vi "NEW_Surge IFSM.vi"() -> ()   [LabVIEW 2019]
uses:
  <vilib>/Utility/NIReport.llb/Report Type.ctl
  <vilib>/Utility/NIReport.llb/NI_report.lvclass
  <vilib>/Utility/NIReport.llb/NI_ReportGenerationCore.lvlib
  <vilib>/Utility/NIReport.llb/Excel/NI_Excel.lvclass
panel:
  in  "REQUEST NUMBER":i32
  out "STEP 8":bool
  out "STEP 7":bool
  out "STEP 6":bool
  out "STEP 5":bool
  in  "START Button":bool
  out "STEP 4":bool
  out "STEP 3":bool
  out "STEP 2":bool
  out "STEP 1":bool
  in  "FILE PATH":path
  # "DATA SUMMARY FOR SURGE IFSM"
  # "OPEN EXCEL FILE"
  # "RUN MACRO INTO EXCEL FILE"
  # "Create New Sheet named (Request Number_Surge_IFSM)"
  # "Create Table named (\"Last  Good Pass\")"
  # "Create New Sheet and Table named (\"Summary Table\")"
  # "Move All Tabs into a new Excel Workbook"
  # "SAVE EXCEL FILE"
  # "FINISH"
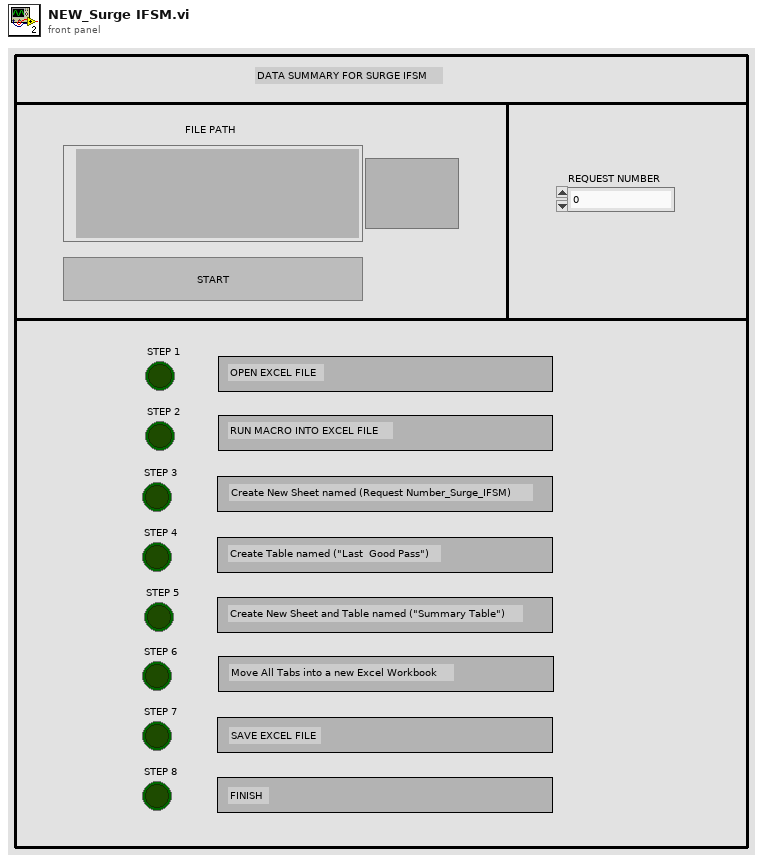
[diagram p1: front panel]
types:
  T1 = enum16{"maximized", "minimized", "normal", "no change"}
  T2 = typedef "NI_ReportGenerationCore.lvlib/Report Type.ctl" = enum16{"HTML", "Word", "Excel"}
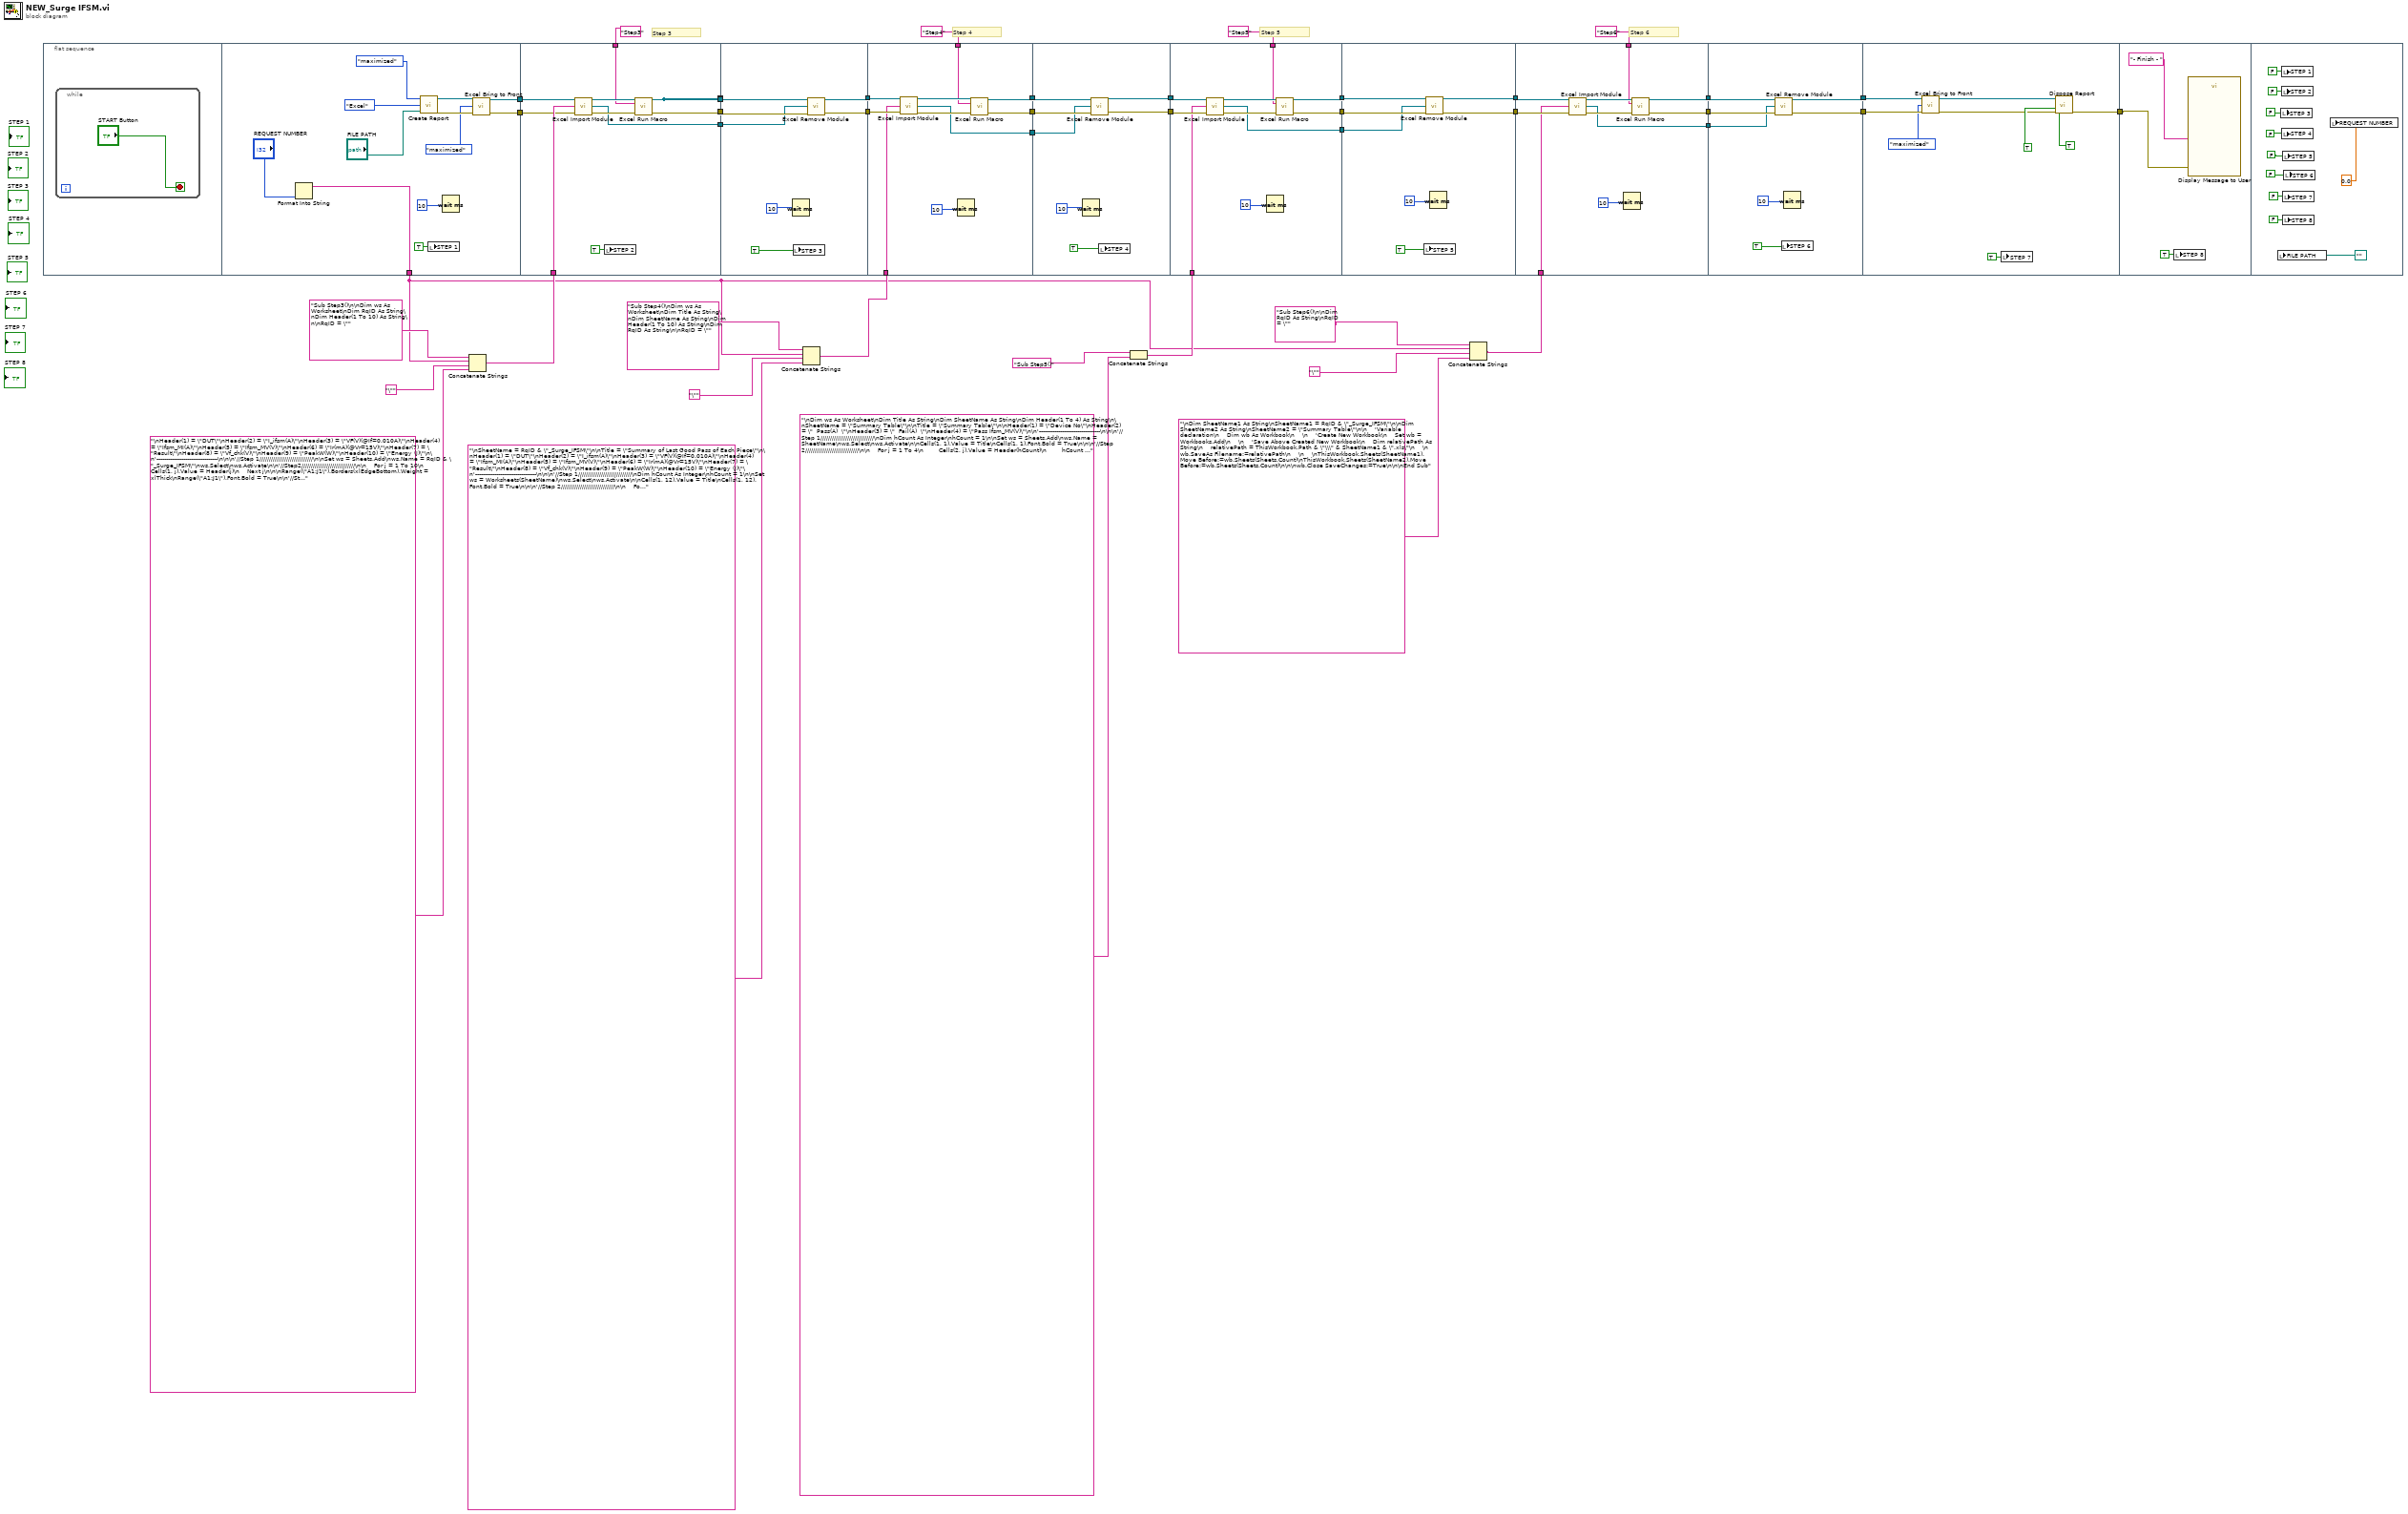
[diagram p0: block diagram]
diagram:
  # "Step 3"
  # "Step 6"
  # "Step 5"
  # "Step 4"
  n1 = flat-sequence {
    tunnel: [w50] -> w38
    tunnel: [w49] -> w37
    tunnel: [w46] -> w1
    tunnel: [w65] -> w43
    tunnel: [w63] -> w42
    tunnel: "Step3" ("macro name") -> [w64]
    tunnel: [w63] -> w40
    tunnel: [w62] -> w39
    tunnel: w20 -> [w60]
    tunnel: w38 -> [w59]
    tunnel: w37 -> [w58]
    tunnel: w43 -> [w73]
    tunnel: [w71] -> w36
    tunnel: w42 -> [_]
    tunnel: [w72] -> w35
    tunnel: w40 -> [w74]
    tunnel: w39 -> [w70]
    tunnel: w36 -> [w81]
    tunnel: [w79] -> w34
    tunnel: w35 -> [w84]
    tunnel: [w82] -> w33
    tunnel: "Step4" ("macro name") -> [w78]
    tunnel: [w77] -> w21
    tunnel: w3 -> [w76]
    tunnel: w34 -> [w90]
    tunnel: w33 -> [w87]
    tunnel: [w89] -> w23
    tunnel: [w88] -> w22
    tunnel: w21 -> [w86]
    tunnel: [w96] -> w32
    tunnel: [w99] -> w31
    tunnel: w23 -> [w98]
    tunnel: w22 -> [w101]
    tunnel: "Step5" ("macro name") -> [w95]
    tunnel: [w94] -> w18
    tunnel: w17 -> [w93]
    tunnel: w32 -> [w107]
    tunnel: [w106] -> w28
    tunnel: w31 -> [w104]
    tunnel: [w105] -> w26
    tunnel: w18 -> [w103]
    tunnel: w28 -> [w118]
    tunnel: [w116] -> w27
    tunnel: w26 -> [w115]
    tunnel: [w113] -> w25
    tunnel: "Step6" ("macro name") -> [w112]
    tunnel: [w111] -> w15
    tunnel: w14 -> [w110]
    tunnel: w27 -> [w124]
    tunnel: [w123] -> w30
    tunnel: w25 -> [w122]
    tunnel: [w121] -> w29
    tunnel: w15 -> [w120]
    tunnel: w30 -> [w129]
    tunnel: w29 -> [w130]
    tunnel: [w133] -> w44
    tunnel: w44 -> [w135]
    frame #0 {
      n2 = while {
        stop <- "START Button" stop-if-true
      }
    }
    frame #1 {
      n3 = Format Into String("REQUEST NUMBER") -> (resulting string=w46:string)  [unwired: 3 in, 1 out]
      n4 = call <vilib>:"Create Report.vi"("window state (normal)"=T1."maximized", "report type"=Report_Type."Excel", "template (empty)"="FILE PATH") -> ("report out"=w53:refnum<class "NI_report.lvclass">, "error out"=w54:errorcluster)  [unwired: 11 in]
      n5 = local write "STEP 1"(TRUE ("STEP 1")) -> ()
      n6 = Wait (ms)(milliseconds to wait=u32 10 ("millisecond timer value")) -> ()  [unwired: 1 out]
      n7 = call <vilib>:"Excel Bring to Front.vi"("report in"=w53, "window state (maximized)"=enum16{"maximized", "minimized", "normal"}."maximized", "error in (no error)"=w54) -> ("report out"=w50:refnum<class "NI_report.lvclass">, "error out"=w49:errorcluster)  [unwired: 11 in]
    }
    frame #2 {
      n8 = call <vilib>:"Excel Import Module.vi"("report in"=w59, "module code (\"\")"=w60, "error in (no error)"=w58) -> ("report out"=w67:refnum<class "NI_report.lvclass">, "module reference"=w62:refnum<k7>, "error out"=w66:errorcluster)  [unwired: 10 in]
      n9 = local write "STEP 2"(TRUE ("STEP 2")) -> ()
      n10 = call <vilib>:"Excel Run Macro.vi"("report in"=w67, "macro name"=w64, "error in (no error)"=w66) -> ("report out"=w63:refnum<class "NI_report.lvclass">, "error out"=w65:errorcluster)  [unwired: 10 in, 1 out]
    }
    frame #3 {
      n11 = Wait (ms)(milliseconds to wait=u32 10 ("millisecond timer value")) -> ()  [unwired: 1 out]
      n12 = local write "STEP 3"(TRUE) -> ()
      n13 = call <vilib>:"Excel Remove Module.vi"("report in"=w74, "module reference"=w70, "error in (no error)"=w73) -> ("report out"=w72:refnum<class "NI_report.lvclass">, "error out"=w71:errorcluster)  [unwired: 11 in]
    }
    frame #4 {
      n14 = call <vilib>:"Excel Import Module.vi"("report in"=w84, "module code (\"\")"=w76, "error in (no error)"=w81) -> ("report out"=w83:refnum<class "NI_report.lvclass">, "module reference"=w77:refnum<k7>, "error out"=w80:errorcluster)  [unwired: 10 in]
      n15 = Wait (ms)(milliseconds to wait=u32 10 ("millisecond timer value")) -> ()  [unwired: 1 out]
      n16 = call <vilib>:"Excel Run Macro.vi"("report in"=w83, "macro name"=w78, "error in (no error)"=w80) -> ("report out"=w82:refnum<class "NI_report.lvclass">, "error out"=w79:errorcluster)  [unwired: 10 in, 1 out]
    }
    frame #5 {
      n17 = Wait (ms)(milliseconds to wait=u32 10 ("millisecond timer value")) -> ()  [unwired: 1 out]
      n18 = call <vilib>:"Excel Remove Module.vi"("report in"=w87, "module reference"=w86, "error in (no error)"=w90) -> ("report out"=w88:refnum<class "NI_report.lvclass">, "error out"=w89:errorcluster)  [unwired: 11 in]
      n19 = local write "STEP 4"(TRUE) -> ()
    }
    frame #6 {
      n20 = call <vilib>:"Excel Import Module.vi"("report in"=w101, "module code (\"\")"=w93, "error in (no error)"=w98) -> ("report out"=w100:refnum<class "NI_report.lvclass">, "module reference"=w94:refnum<k7>, "error out"=w97:errorcluster)  [unwired: 10 in]
      n21 = Wait (ms)(milliseconds to wait=u32 10 ("millisecond timer value")) -> ()  [unwired: 1 out]
      n22 = call <vilib>:"Excel Run Macro.vi"("report in"=w100, "macro name"=w95, "error in (no error)"=w97) -> ("report out"=w99:refnum<class "NI_report.lvclass">, "error out"=w96:errorcluster)  [unwired: 10 in, 1 out]
    }
    frame #7 {
      n23 = local write "STEP 5"(TRUE) -> ()
      n24 = call <vilib>:"Excel Remove Module.vi"("report in"=w104, "module reference"=w103, "error in (no error)"=w107) -> ("report out"=w105:refnum<class "NI_report.lvclass">, "error out"=w106:errorcluster)  [unwired: 11 in]
      n25 = Wait (ms)(milliseconds to wait=u32 10 ("millisecond timer value")) -> ()  [unwired: 1 out]
    }
    frame #8 {
      n26 = call <vilib>:"Excel Import Module.vi"("report in"=w115, "module code (\"\")"=w110, "error in (no error)"=w118) -> ("report out"=w114:refnum<class "NI_report.lvclass">, "module reference"=w111:refnum<k7>, "error out"=w117:errorcluster)  [unwired: 10 in]
      n27 = Wait (ms)(milliseconds to wait=u32 10 ("millisecond timer value")) -> ()  [unwired: 1 out]
      n28 = call <vilib>:"Excel Run Macro.vi"("report in"=w114, "macro name"=w112, "error in (no error)"=w117) -> ("report out"=w113:refnum<class "NI_report.lvclass">, "error out"=w116:errorcluster)  [unwired: 10 in, 1 out]
    }
    frame #9 {
      n29 = call <vilib>:"Excel Remove Module.vi"("report in"=w122, "module reference"=w120, "error in (no error)"=w124) -> ("report out"=w121:refnum<class "NI_report.lvclass">, "error out"=w123:errorcluster)  [unwired: 11 in]
      n30 = local write "STEP 6"(TRUE) -> ()
      n31 = Wait (ms)(milliseconds to wait=u32 10 ("millisecond timer value")) -> ()  [unwired: 1 out]
    }
    frame #10 {
      n32 = call <vilib>:"Excel Bring to Front.vi"("report in"=w130, "window state (maximized)"=enum16{"maximized", "minimized", "normal"}."maximized", "error in (no error)"=w129) -> ("report out"=w127:refnum<class "NI_report.lvclass">, "error out"=w126:errorcluster)  [unwired: 11 in]
      n33 = local write "STEP 7"(TRUE ("STEP 3")) -> ()
      n34 = call-dynamic "Dispose Report.vi"("report in"=w127, "save changes? (F)"=TRUE, "error in (no error)"=w126, "close report? (T)"=TRUE) -> ("error out"=w133:errorcluster)  [unwired: 11 in]
    }
    frame #11 {
      n35 = local write "STEP 8"(TRUE ("STEP 4")) -> ()
      n36 = call "Display Message to User"("error in (no error)"=w135, "Message"="- Finish - ") -> ()  [unwired: 8 in, 2 out]
    }
    frame #12 {
      n37 = local write "FILE PATH"(path "" ("FILE PATH")) -> ()
      n38 = local write "STEP 3"(FALSE) -> ()
      n39 = local write "STEP 1"(FALSE ("STEP 1")) -> ()
      n40 = local write "STEP 2"(FALSE ("STEP 2")) -> ()
      n41 = local write "STEP 4"(FALSE) -> ()
      n42 = local write "STEP 5"(FALSE) -> ()
      n43 = local write "STEP 7"(FALSE ("STEP 3")) -> ()
      n44 = local write "STEP 8"(FALSE ("STEP 4")) -> ()
      n45 = local write "STEP 6"(FALSE) -> ()
      n46 = local write "REQUEST NUMBER"(0.0 ("REQUEST NUMBER")) -> ()
    }
  }
  n47 = Concatenate Strings("Sub Step3()\n\nDim ws As Worksheet\nDim RqID As String\nDim Header(1 To 10) As String\n\nRqID = \"" ("string"), w1, "\"" ("string"), "\nHeader(1) = \"DUT\"\nHeader(2) = \"I_ifsm(A)\"\nHeader(3) = \"VF(V)(@If=0.010A)\"\nHeader(4) = \"Ifsm_MI(A)\"\nHeader(5) = \"Ifsm_MV(V)\"\nHeader(6) = \"Ir(mA)(@Vr=15V)\"\nHeader(7) = \"Result\"\nHeader(8) = \"Vf_chk(V)\"\nHeader(9) = \"PeakW(W)\"\nHeader(10) = \"Energy (J)\"\n\n'--------------------------------\n\n\n'//Step 1////////////////////////////\n\nSet ws = Sheets.Add\nws.Name = RqID & \"_Surge_IFSM\"\nws.Select\nws.Activate\n\n'//Step2////////////////////////////\n\n    For j = 1 To 10\n        Cells(1, j).Value = Header(j)\n    Next j\n\n\nRange(\"A1:J1\").Borders(xlEdgeBottom).Weight = xlThick\nRange(\"A1:J1\").Font.Bold = True\n\n'//Step3 to 7////////////////////////////\n\nDim CountFront As Integer\nDim SheetN As Integer\nDim msg As String\nSheetN = (Sheets.Count)\nCountFront = 0\nReDim Status(1 To SheetN) As String\n\n\n    '// Count how many available hastag\n    For j = 1 To SheetN\n            If InStr(1, (Sheets(j).Name), \"#\") = 2 Then\n                Status(j) = j\n                CountFront = CountFront + 1\n            Else\n                Status(j) = 0\n            End If\n    Next j\n\n'// Insert number(string) into array\n    Dim RowResultValue As Integer\n    Dim RowInputValue As Integer\n    Dim DUT As Integer\n    Dim StRange As String\n    Dim StLine As String\n    \n    \n    RowResultValue = 2\n    RowInputValue = 12\n    DUT = 1\n\n    \n    \n    For m = 1 To SheetN\n\n        If Status(m) = 0 Then\n\n        Else\n                    If Sheets(m).Columns(7).Rows(RowInputValue).Value <> \"FAIL\" Then\n                    \n                                Do While Sheets(m).Columns(7).Rows(RowInputValue).Value <> \"FAIL\"\n                                \n                                StRange = \"B\" & RowInputValue & \":J\" & RowInputValue\n                                \n                                ws.Columns(1).Rows(RowResultValue) = DUT\n                                Sheets(m).Range(StRange).Copy ws.Columns(2).Rows(RowResultValue)\n                                \n                                \n                                RowResultValue = RowResultValue + 1\n                                RowInputValue = RowInputValue + 1\n                                Loop\n                    End If\n                    \n                    \n                    \n                    If Sheets(m).Columns(7).Rows(RowInputValue).Value = \"FAIL\" Then\n                   StRange = \"B\" & RowInputValue & \":J\" & RowInputValue\n                    ws.Columns(1).Rows(RowResultValue) = DUT\n                    Sheets(m).Range(StRange).Copy ws.Columns(2).Rows(RowResultValue)\n                    \n                    StLine = \"A\" & RowResultValue & \":J\" & RowResultValue\n                    Range(StLine).Borders(xlEdgeBottom).Weight = xlThick\n                    \n                    RowResultValue = RowResultValue + 1\n                    RowInputValue = RowInputValue + 1\n                    \n                    Else\n                    \n                    MsgBox \" No Fail \"\n                    \n                    End If\n\nDUT = DUT + 1\n                    RowInputValue = 12\n        End If\n\n    \n    \n    \n    Next m\n\nEnd Sub " ("string")) -> (w20:string)
  n48 = Concatenate Strings("Sub Step4()\nDim ws As Worksheet\nDim Title As String\nDim SheetName As String\nDim Header(1 To 10) As String\nDim RqID As String\n\nRqID = \"" ("string"), w1, "\"" ("string"), "\nSheetName = RqID & \"_Surge_IFSM\"\n\nTitle = \"Summary of Last Good Pass of Each Piece\"\n\nHeader(1) = \"DUT\"\nHeader(2) = \"I_ifsm(A)\"\nHeader(3) = \"VF(V)(@If=0.010A)\"\nHeader(4) = \"Ifsm_MI(A)\"\nHeader(5) = \"Ifsm_MV(V)\"\nHeader(6) = \"Ir(mA)(@Vr=15V)\"\nHeader(7) = \"Result\"\nHeader(8) = \"Vf_chk(V)\"\nHeader(9) = \"PeakW(W)\"\nHeader(10) = \"Energy (J)\"\n'--------------------------------\n\n\n'//Step 1////////////////////////////\nDim hCount As Integer\nhCount = 1\n\nSet ws = Worksheets(SheetName)\nws.Select\nws.Activate\n\nCells(1, 12).Value = Title\nCells(1, 12).Font.Bold = True\n\n\n'//Step 2////////////////////////////\n\n    For j = 12 To 21\n        Cells(2, j).Value = Header(hCount)\n        hCount = hCount + 1\n    Next j\n\n\nRange(\"L2:U2\").Borders(xlEdgeBottom).Weight = xlThick\nRange(\"L2:U2\").Font.Bold = True\n\n\n\n'//Step3 to 4////////////////////////////\n\nDim CountFront As Integer\nDim SheetN As Integer\nDim msg As String\nSheetN = (Sheets.Count)\nCountFront = 0\nReDim Status(1 To SheetN) As String\n\n\n    '// Count how many available hastag\n    For j = 1 To SheetN\n            If InStr(1, (Sheets(j).Name), \"#\") = 2 Then\n                Status(j) = j\n                CountFront = CountFront + 1\n            Else\n                Status(j) = 0\n            End If\n    Next j\n\n    'Front Array\n    'ReDim Front(1 To CountFront) As Integer\n    'Dim Chars As String\n\n\n    '// Insert number(string) into array\n    Dim RowResultValue As Integer\n    Dim RowInputValue As Integer\n    Dim DUT As Integer\n    Dim StRange As String\n    Dim StLine As String\n\n\n    RowResultValue = 3\n    RowInputValue = 12\n    DUT = 1\n\n\n\n    For m = 1 To SheetN\n\n        If Status(m) = 0 Then\n\n        Else\n                    If Sheets(m).Columns(7).Rows(RowInputValue).Value <> \"FAIL\" Then\n\n                                Do While Sheets(m).Columns(7).Rows(RowInputValue).Value <> \"FAIL\"\n\n'                                StRange = \"B\" & RowInputValue & \":J\" & RowInputValue\n'\n'                                ws.Columns(1).Rows(RowResultValue) = DUT\n'                                Sheets(m).Range(StRange).Copy ws.Columns(2).Rows(RowResultValue)\n\n'\n'                                RowResultValue = RowResultValue + 1\n                                RowInputValue = RowInputValue + 1\n                                Loop\n                    End If\n\n\n\n                    If Sheets(m).Columns(7).Rows(RowInputValue).Value = \"FAIL\" Then\nStRange = \"B\" & (RowInputValue - 1) & \":J\" & (RowInputValue - 1)\n                    ws.Columns(12).Rows(RowResultValue) = DUT\n                    Sheets(m).Range(StRange).Copy ws.Columns(13).Rows(RowResultValue)\n\nRowResultValue = RowResultValue + 1\n                    RowInputValue = RowInputValue + 1\n\n                    Else\n\n                    MsgBox \" No Fail \"\n\n                    End If\n\nDUT = DUT + 1\n                    RowInputValue = 12\n        End If\n\n\n\n\n    Next m\n\nEnd Sub" ("string")) -> (w3:string)
  n49 = Concatenate Strings("Sub Step5()" ("string"), "\nDim ws As Worksheet\nDim Title As String\nDim SheetName As String\nDim Header(1 To 4) As String\n\nSheetName = \"Summary Table\"\n\nTitle = \"Summary Table\"\n\nHeader(1) = \"Device No\"\nHeader(2) = \"  Pass(A)  \"\nHeader(3) = \"  Fail(A)  \"\nHeader(4) = \"Pass Ifsm_MV(V)\"\n\n'--------------------------------\n\n\n'//Step 1////////////////////////////\nDim hCount As Integer\nhCount = 1\n\nSet ws = Sheets.Add\nws.Name = SheetName\nws.Select\nws.Activate\n\nCells(1, 1).Value = Title\nCells(1, 1).Font.Bold = True\n\n\n'//Step 2////////////////////////////\n\n    For j = 1 To 4\n        Cells(2, j).Value = Header(hCount)\n        hCount = hCount + 1\n    Next j\n\n\nRange(\"A2:D2\").Borders(xlEdgeBottom).Weight = xlThick\nRange(\"A2:D2\").Borders.LineStyle = xlContinuous\nRange(\"A2:D2\").Font.Bold = True\nRange(\"A2:D2\").Columns.AutoFit\nRange(\"A2:D2\").Interior.ColorIndex = 6 'Yellow\n\n'//Step3 to 4////////////////////////////\n\nDim CountFront As Integer\nDim SheetN As Integer\nDim msg As String\nSheetN = (Sheets.Count)\nCountFront = 0\nReDim Status(1 To SheetN) As String\n\n\n    '// Count how many available hastag\n    For j = 1 To SheetN\n            If InStr(1, (Sheets(j).Name), \"#\") = 2 Then\n                Status(j) = j\n                CountFront = CountFront + 1\n            Else\n                Status(j) = 0\n            End If\n    Next j\n\n'// Insert number(string) into array\n    Dim RowResultValue As Integer\n    Dim RowInputValue As Integer\n    Dim DUT As Integer\n'    Dim StRange As String\n    Dim StPass As String\n    Dim StFail As String\n    Dim StIfsmPass As String\n    Dim St4Border As String\n'    Dim StLine As String\n\n\n    RowResultValue = 3\n    RowInputValue = 12\n    DUT = 1\n\n\n\n    For m = 1 To SheetN\n\n        If Status(m) = 0 Then\n\n        Else\n                    If Sheets(m).Columns(7).Rows(RowInputValue).Value <> \"FAIL\" Then\n\n                                Do While Sheets(m).Columns(7).Rows(RowInputValue).Value <> \"FAIL\"\n                                RowInputValue = RowInputValue + 1\n                                Loop\n                    End If\n\n\n\n                    If Sheets(m).Columns(7).Rows(RowInputValue).Value = \"FAIL\" Then\n\nStPass = \"B\" & (RowInputValue - 1)\n                    StFail = \"B\" & (RowInputValue)\n                    StIfsmPass = \"E\" & (RowInputValue - 1)\n                    St4Border = \"A\" & (RowResultValue) & \":D\" & (RowResultValue)\n\n                    ws.Columns(1).Rows(RowResultValue) = DUT 'DUT\n                    ws.Columns(2).Rows(RowResultValue) = Sheets(m).Range(StPass) 'PASS\n                    ws.Columns(3).Rows(RowResultValue) = Sheets(m).Range(StFail) 'FAIL\n                    ws.Columns(4).Rows(RowResultValue) = Sheets(m).Range(StIfsmPass) 'Pass Ifsm_MV(V)\n                    \n                    ws.Range(St4Border).Borders.LineStyle = xlContinuous\n\nRowResultValue = RowResultValue + 1\n                    RowInputValue = RowInputValue + 1\n\n                    Else\n\n                    MsgBox \" No Fail \"\n\n                    End If\n\nDUT = DUT + 1\n                    RowInputValue = 12\n        End If\n\n\n\n\n    Next m\n\nEnd Sub" ("string")) -> (w17:string)
  n50 = Concatenate Strings("Sub Step6()\n\nDim RqID As String\nRqID = \"" ("string"), w1, "\"" ("string"), "\nDim SheetName1 As String\nSheetName1 = RqID & \"_Surge_IFSM\"\n\nDim SheetName2 As String\nSheetName2 = \"Summary Table\"\n\n    'Variable declaration\n    Dim wb As Workbook\n    \n    'Create New Workbook\n    Set wb = Workbooks.Add\n    \n    'Save Above Created New Workbook\n    Dim relativePath As String\n    relativePath = ThisWorkbook.Path & \"\\\" & SheetName1 & \".xls\"\n    \n    wb.SaveAs Filename:=relativePath\n    \n    \nThisWorkbook.Sheets(SheetName1).Move Before:=wb.Sheets(Sheets.Count)\nThisWorkbook.Sheets(SheetName2).Move Before:=wb.Sheets(Sheets.Count)\n\n\nwb.Close SaveChanges:=True\n\n\nEnd Sub" ("string")) -> (w14:string)
